vi "DtOLReadMultiple1DU16.vi"(6 "Buffer size":u32, 7 "OnlyReadAvailable":bool, 8 "error in (no error)":errorcluster, 9 "Timeout":dbl=10.0, 10 "Samples Per Channel":i32=-1, 11 "Task in":i32) -> (0 "error out":errorcluster, 1 "Num Samples Read":u32, 2 "1D Data out":u16[](array[numeric]), 3 "Task out":i32)   [LabVIEW 2016]
doc: "Reads multiple samples from a single virtual channel of a task you specify, and returns the data as a one-dimensional array of unsigned, 16-bit numbers. This VI is typically used with analog input tasks that use the DtOLTiming (Input - Set Timing) VI."
uses:
  <userlib>/LV-Link3/DtLvLink.lvlib
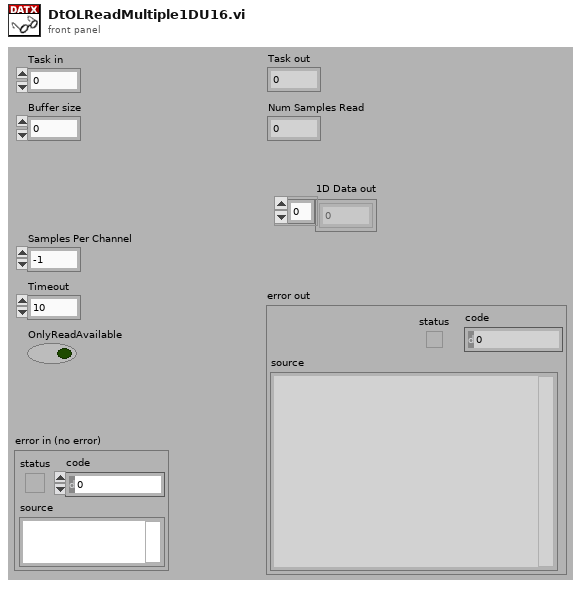
[diagram p1: front panel]
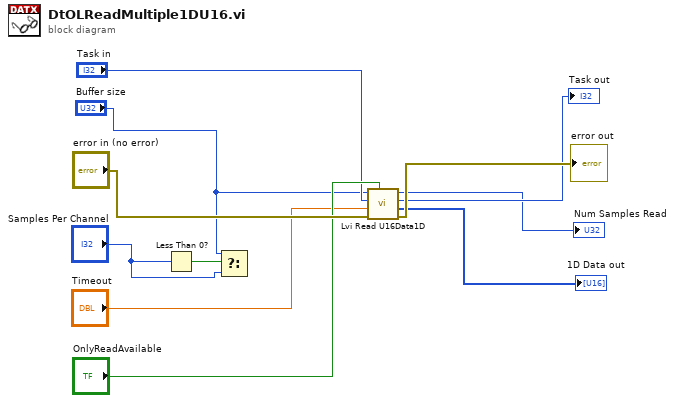
[diagram p0: block diagram]
diagram:
  n1 = Less Than 0?(x="Samples Per Channel") -> (x < 0?=w6:bool)
  n2 = Select(t="Buffer size", s=w6, f="Samples Per Channel") -> ()  [unwired: 1 out]
  n3 = call <userlib>:"Lvi Read U16Data1D.vi"("OnlyReadAvailable"="OnlyReadAvailable", "error in (no error)"="error in (no error)", "timeout"="Timeout", "TaskRef"="Task in", "DataBufSize"="Buffer size") -> ("error out"=→"error out":errorcluster, "DataBuf"=→"1D Data out":u16[], "TaskRef out"=→"Task out":i32, "DataBufSize out"=→"Num Samples Read":u32)  [unwired: 2 in, 1 out]
